vi "Set Waveform Type.vi"(8 "error in (no error)":errorcluster, 9 "2nd Waveform (0: None)":u32(ring) items=["None", "Sine", "Triangle", "Square", "Truncated Sine"], 10 "1st Waveform (0: None)":u32(ring) items=["None", "Sine", "Triangle", "Square", "Truncated Sine"], 11 "VISA resource name":refnum<visa-resource-name>) -> (0 "error out":errorcluster, 3 "VISA resource name out":refnum<visa-resource-name>)   [LabVIEW 2014, in "Fluke 5XXX Series Multicalibrators.lvlib"]
doc: "This VI sets the waveforms for ac outputs. If the Calibrator is sourcing one output, one parameter is required. If the Calibrator is sourcing two outputs, two parameters are required or one parameter to set the waveform to both outputs. Waveform choices are SINE (sinewave), TRI (trianglewave), SQUARE (squarewave), TRUNCS (truncated sinewave), or NONE (waveform does not apply).\n\nNote:\n\nThis VI is available only for instrument models 5500A and 5520A."
uses:
  Fluke 5XXX Series Multicalibrators.lvlib
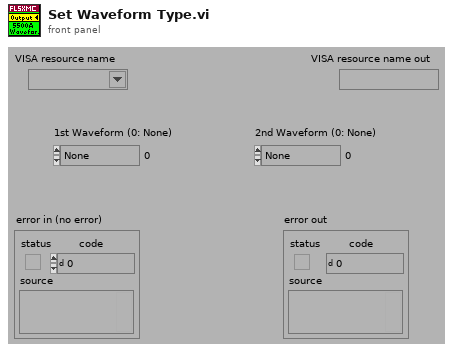
[diagram p1: front panel]
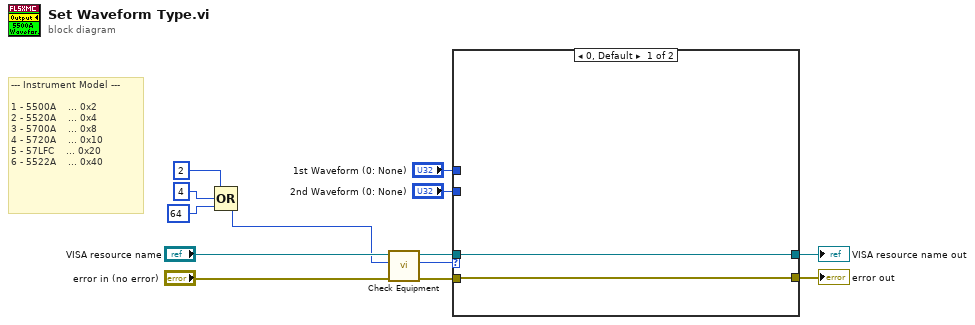
[diagram p0: block diagram]
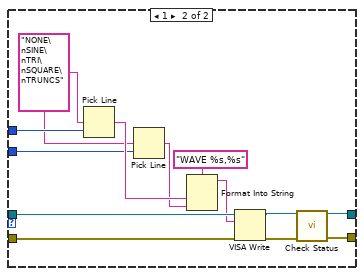
[diagram p2: hidden frame]
diagram:
  # "--- Instrument Model ---\n\n1 - 5500A    ... 0x2\n2 - 5520A    ... 0x4\n3 - 5700A    ... 0x8\n4 - 5720A    ... 0x10\n5 - 57LFC    ... 0x20\n6 - 5522A    ... 0x40"
  n1 = Compound Arithmetic op=OR(2 ("Numeric"), 4 ("Numeric"), 64 ("Numeric")) -> (w4:i32)
  n2 = call "Check Equipment.vi"("error in (no error)"="error in (no error)", "Bit Mask"=w4, "VISA resource name"="VISA resource name") -> ("error out"=w13:errorcluster, "Present?"=w12:u32, "VISA resource name out"=w11:refnum<visa-resource-name>)  [unwired: 6 in]
  n3 = case shown="0, Default" w12 {
    tunnel: [w14 w23] -> w9
    tunnel: w13 -> [w15 w28]
    tunnel: w11 -> [w14 w27]
    tunnel: [w15 w26] -> w10
    tunnel: "1st Waveform (0: None)" -> [_ w18]
    tunnel: "2nd Waveform (0: None)" -> [_ w17]
    frame 0, Default {
    }
    frame 1 {
      w16 = "NONE\nSINE\nTRI\nSQUARE\nTRUNCS"
      n4 = Pick Line(multi-line string=w16, line index=w18) -> (output string=w20:string)  [unwired: 1 in]
      n5 = Pick Line(multi-line string=w16, line index=w17) -> (output string=w19:string)  [unwired: 1 in]
      n6 = Format Into String(format string="WAVE %s,%s", w20, w19) -> (resulting string=w21:string)  [unwired: 2 in, 1 out]
      n7 = VISA Write(VISA resource name=w27, write buffer=w21, error in (no error)=w28) -> (VISA resource name out=w24:refnum<visa-resource-name>, error out=w25:errorcluster)  [unwired: 1 out]
      n8 = call "Check Status.vi"("VISA resource name"=w24, "error in (no error)"=w25) -> ("VISA resource name out"=w23:refnum<visa-resource-name>, "error out"=w26:errorcluster)  [unwired: 12 in]
    }
  }
  "VISA resource name out" <- w9
  "error out" <- w10
